vi "Encrypt Letter (Var).vi"(8 "error in":errorcluster, 10 "letter":string, 11 "Variant in":variant) -> (0 "error out":errorcluster, 2 "encrypted letter":string, 3 "Variant out":variant)   [LabVIEW 2015]
uses:
  Letter/Letter.lvclass
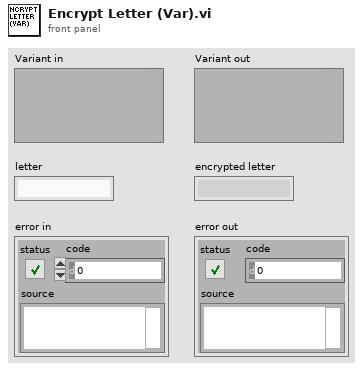
[diagram p1: front panel]
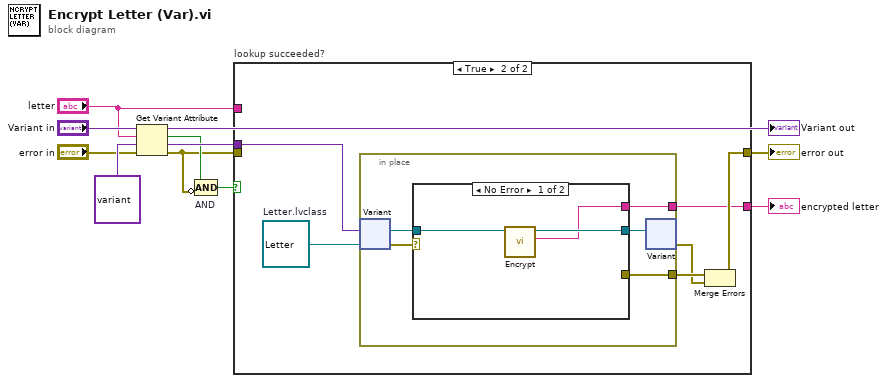
[diagram p0: block diagram]
diagram:
  n1 = Get Variant Attribute(Variant="Variant in", name="letter", default value (empty Variant)=variant, error in="error in") -> (duplicate Variant=→"Variant out":variant, found=w7:bool, value=w8:variant, error out=w6:errorcluster)
  n2 = Compound Arithmetic op=AND "AND"(w7, invert w6) -> (w5:bool)
  n3 = case "lookup succeeded?" shown="True" w5 {
    tunnel: w8 -> [_ w19]
    tunnel: w6 -> [w13 _]
    tunnel: [w13 w15] -> w4
    tunnel: [w12 w14] -> w2
    tunnel: "letter" -> [w12 _]
    frame False {
      # "Output original character"
    }
    frame True {
      w18 = refnum<class "Letter.lvclass"> refnum  # Letter.lvclass
      n4 = in-place {
        in-place-border: [w21] -> w17
        in-place-border: [w20] -> w14
        n5 = in-place-variant #1(w19, w18) -> (w22:refnum<class "Letter.lvclass">, w24:errorcluster)
        n6 = case shown="No Error" w24 {
          selector: w24 -> [_ w28]
          tunnel: [w26 w29] -> w23
          tunnel: w22 -> [w27 w29]
          tunnel: [_ w28] -> w21
          tunnel: [w25 _] -> w20
          frame No Error {
            n7 = call "Encrypt.vi"("Letter in"=w27) -> ("letter"=w25:string, "Letter out"=w26:refnum<class "Letter.lvclass">)  [unwired: 9 in]
          }
          frame Error {
          }
        }
        n8 = in-place-variant #1(w23) -> (w16:errorcluster)  [unwired: 1 out]
      }
      n9 = Merge Errors(w17, w16) -> (w15:errorcluster)
    }
  }
  "error out" <- w4
  "encrypted letter" <- w2
